vi "Init.vi"(3 "Container State":T3, 4 "Previous State":variant, 5 "Previous Version":T2) -> (2 "Current State":T1)   [LabVIEW 2014, in "XListGraph.lvlib" / "XListGraph.xctl"]
uses:
  XListGraph.xctl
  State.ctl
  Support/def-XListGraphOper.ctl
  <vilib>/_xctls/Container State.ctl
  <vilib>/_xctls/Version.ctl
  <vilib>/_xctls/XControlSupport.lvlib
panel:
  in  "Default Indicator State":T1
  in  "Default Control State":T1
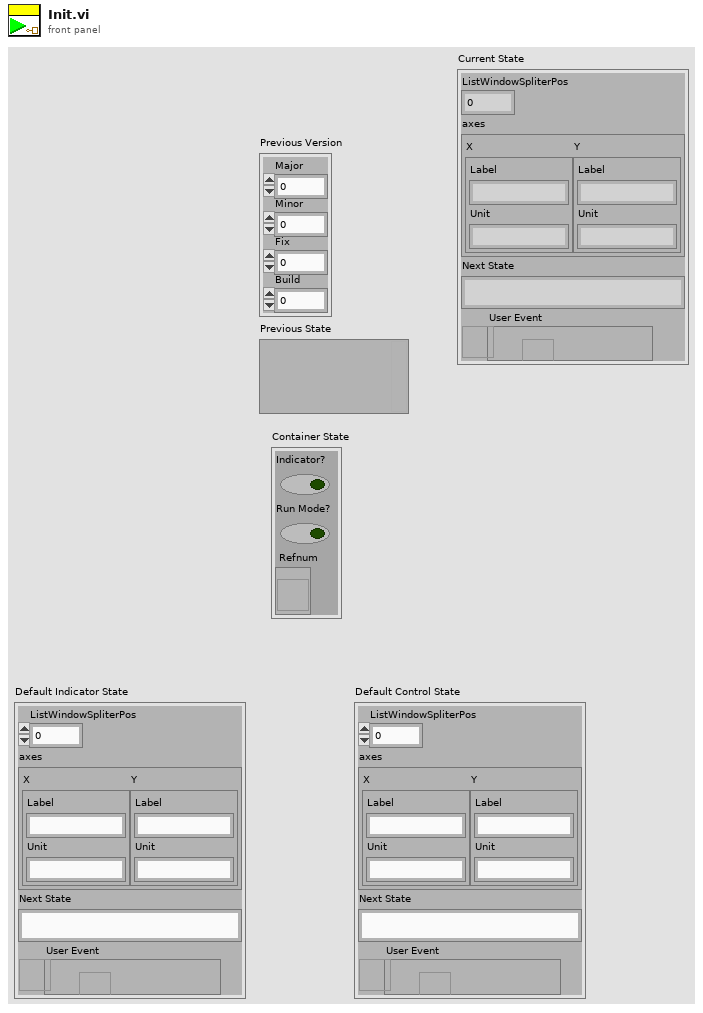
[diagram p1: front panel]
types:
  T1 = typedef "XListGraph.lvlib/XListGraph.xctl/State.ctl" = cluster{"ListWindowSpliterPos":i32, "axes":cluster{"X":cluster{"Label":string, "Unit":string}, "Y":cluster{"Label":string, "Unit":string}}, "Next State":string, "User Event":refnum<user-event>}
  T2 = typedef "XControlSupport.lvlib/Version.ctl" = cluster{"Major":u16, "Minor":u16, "Fix":u16, "Build":u16}
  T3 = typedef "XControlSupport.lvlib/Container State.ctl" = cluster{"Indicator?":bool, "Run Mode?":bool, " Refnum":refnum<vi>}
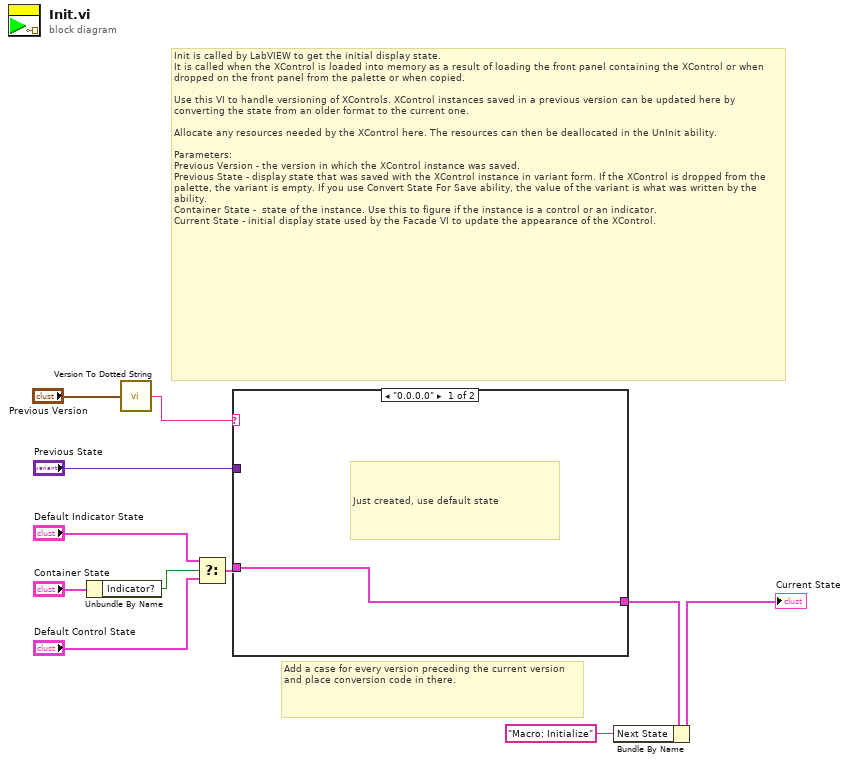
[diagram p0: block diagram]
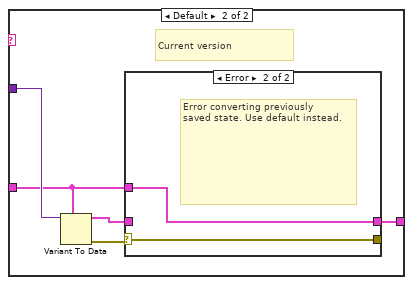
[diagram p2: hidden frame]
diagram:
  # "Add a case for every version preceding the current version and place conversion code in there."
  # "Init is called by LabVIEW to get the initial display state.\nIt is called when the XControl is loaded into memory as a result of loading the front panel containing the XControl or when dropped on the front panel from the palette or when copied.\n\nUse this VI to handle versioning of XControls. XControl instances saved in a previous version can be updated here by converting the state from an older format to the current one.\n\nAllocate any resources needed by the XControl here. The resources can then be deallocated in the UnInit ability.\n\nParameters:\nPrevious Version - the version in which the XControl instance was saved.\nPrevious State - display state that was saved with the XControl instance in variant form. If the XControl is dropped from the palette, the variant is empty. If you use Convert State For Save ability, the value of the variant is what was written by the ability. \nContainer State -  state of the instance. Use this to figure if the instance is a control or an indicator.\nCurrent State - initial display state used by the Facade VI to update the appearance of the XControl."
  n1 = Unbundle By Name("Container State") -> ("Indicator?"=w6:bool)
  n2 = call <vilib>:"Version To Dotted String.vi"("Version"="Previous Version") -> ("String Version"=w3:string)
  n3 = Select(t="Default Indicator State", s=w6, f="Default Control State") -> (s? t:f=w5:T1)
  n4 = case shown="\"0.0.0.0\"" w3 {
    tunnel: "Previous State" -> [_ w17]
    tunnel: [w12 w13] -> w10
    tunnel: w5 -> [w12 w14]
    frame "0.0.0.0" {
      # "Just created, use default state"
    }
    frame Default {
      # "Current version"
      n5 = Variant To Data(type=w14, Variant=w17) -> (data=w15:T1, error out=w16:errorcluster)  [unwired: 1 in]
      n6 = case shown="Error" w16 {
        selector: w16 -> [w19 w20]
        tunnel: w15 -> [w18 _]
        tunnel: [w18 w21] -> w13
        tunnel: w14 -> [_ w21]
        tunnel: [w19 w20] -> _
        frame No Error {
        }
        frame Error {
          # "Error converting previously \nsaved state. Use default instead."
        }
      }
    }
  }
  n7 = Bundle By Name(cluster=w10, "Next State"="Macro: Initialize") -> (→"Current State":T1)
